vi "Save Button Info.vi"(8 "error in":errorcluster, 10 "control info":T1[](array[typedef]) {"Boolean Type" items=["N/A", "FAB--icon--rounded", "outline--icon--rectangular", "outline--icon--rounded", "outline--text--rectangular", "outline--text--rounded", "nooutline--icon--rectangular", "nooutline--icon--rectangular--40x40", "nooutline--icon--rounded", "nooutline--text--rectangular", "nooutline--text--rounded", "tonal--icon--rectangular", "tonal--icon--rounded", "tonal--text--rectangular", "tonal--text--rounded", "filled--icon--rectangular", "filled--icon--rounded", "filled--text--rectangular", "filled--text--rounded"]; "UI Theme Level" items=["N/A", "Primary", "Secondary", "Tertiary", "Error", "Primary Fixed", "Secondary Fixed", "Tertiary Fixed", "Label Only", "No Change"]}, 11 "map in":map{string, refnum<vi>}(c390)) -> (0 "error out":errorcluster)   [LabVIEW 2021]
doc: "This VI will save all of the updated tag data for the controls in the VI reference.\n\n<b>Code Developed By:</b>\nTechnology Service Corporation\nwww.tsc.com/atcs\n\nDeveloper:\nDaniel Coons"
uses:
  control info.ctl
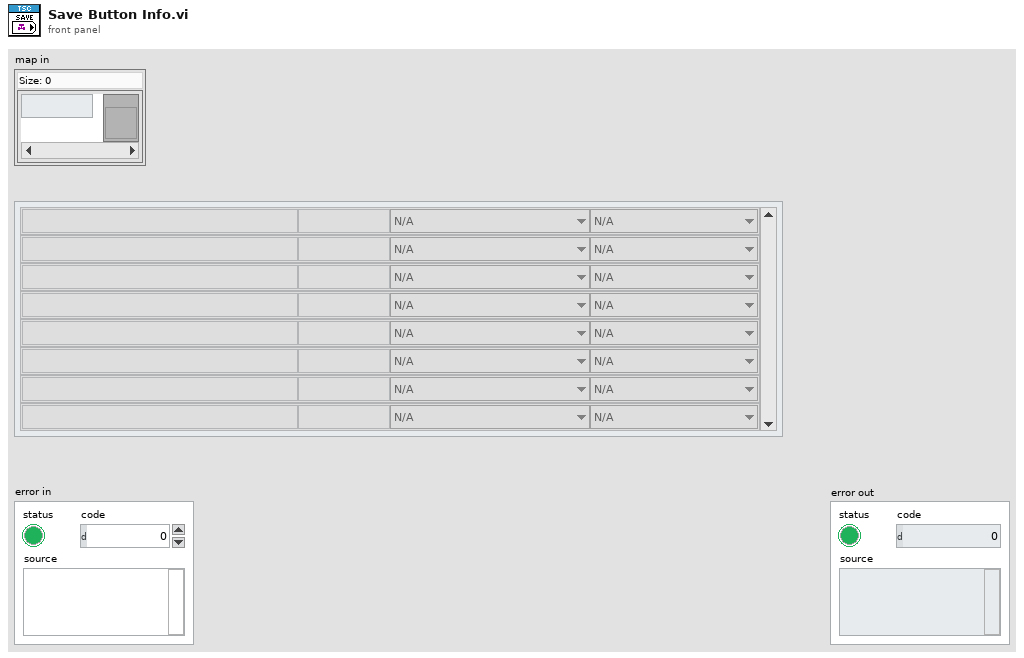
[diagram p1: front panel]
types:
  T1 = typedef "control info.ctl" = cluster{"label":string, "control type":string, "UI Theme Level":u16, "Boolean Type":u16}
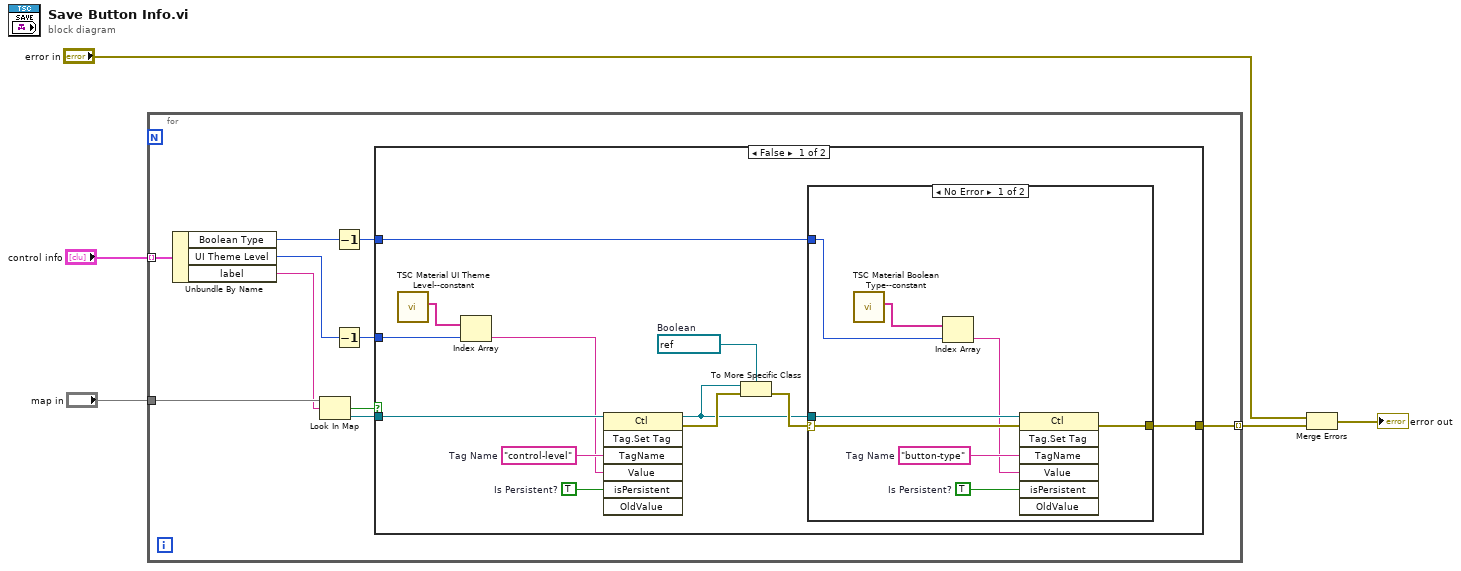
[diagram p0: block diagram]
diagram:
  n1 = for {
    tunnel: "map in" -> [w15]
    tunnel: "control info" -> [w14] mode=indexing
    tunnel: [w8] -> w3 mode=indexing
    n2 = Unbundle By Name(w14) -> ("Boolean Type"=w9:u16, "UI Theme Level"=w10:u16, "label"=w13:string)
    n3 = Look In Map(map=w15, key=w13) -> (key not found?=w12:bool, value=w11:refnum<vi>)  [unwired: 1 in]
    n4 = Decrement(x=w9) -> (x-1=w6:u16)
    n5 = Decrement(x=w10) -> (x-1=w7:u16)
    n6 = case shown="False" w12 {
      tunnel: w11 -> [w23 _]
      tunnel: w7 -> [w26 _]
      tunnel: w6 -> [w16 _]
      tunnel: [w17 _] -> w8
      frame False {
        w20 = refnum<vi> refnum  # Boolean
        w24 = TRUE  # Is Persistent?
        w25 = "control-level"  # Tag Name
        n7 = call "TSC Material UI Theme Level--constant.vi"() -> ("UI theme levels"=w27:string[])  [unwired: 11 in]
        n8 = Index Array(array=w27, index=w26) -> (element=w22:string)
        n9 = invoke class="Ctl" method="Tag.Set Tag"(reference=w23, "TagName"=w25, "Value"=w22, "isPersistent"=w24) -> (reference out=w18:refnum<vi>, error out=w21:errorcluster)  [unwired: 3 in, 5 out]
        n10 = To More Specific Class(target class=w20, reference=w18, error in=w21) -> (error out=w19:errorcluster)  [unwired: 1 out]
        n11 = case shown="No Error" w19 {
          selector: w19 -> [w34 _]
          tunnel: w18 -> [w35 _]
          tunnel: [w33 _] -> w17
          tunnel: w16 -> [w29 _]
          frame No Error {
            w31 = TRUE  # Is Persistent?
            w32 = "button-type"  # Tag Name
            n12 = call "TSC Material Boolean Type--constant.vi"() -> ("boolean types"=w30:string[])  [unwired: 11 in]
            n13 = Index Array(array=w30, index=w29) -> (element=w28:string)
            n14 = invoke class="Ctl" method="Tag.Set Tag"(reference=w35, error in=w34, "TagName"=w32, "Value"=w28, "isPersistent"=w31) -> (error out=w33:errorcluster)  [unwired: 2 in, 6 out]
          }
          frame Error {
          }
        }
      }
      frame True {
      }
    }
  }
  n15 = Merge Errors("error in", w3) -> (→"error out":errorcluster)
